vi "Create.vi"(8 "error in (no error)":errorcluster, 10 "EDVR":refnum<data-value>) -> (0 "error out":errorcluster, 3 "Stream":refnum<data-value>)   [LabVIEW 2020, in "g_ar_toolkit.capture.lvlib" / "CameraStream.lvclass"]
uses:
  CameraStream.lvclass
  CameraStream.lvclass/CameraStream.ctl
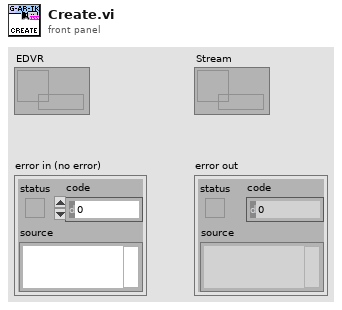
[diagram p1: front panel]
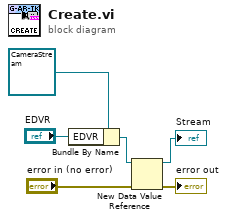
[diagram p0: block diagram]
diagram:
  n1 = Bundle By Name(cluster=refnum<class "CameraStream.lvclass"> refnum ("g_ar_toolkit.lvlib:CameraStream.lvclass"), "EDVR"="EDVR") -> (w2:refnum<class "CameraStream.lvclass">)
  n2 = New Data Value Reference(data value=w2, error in="error in (no error)") -> (data value reference=→"Stream":refnum<data-value>, error out=→"error out":errorcluster)
